vi "3.vi"(8 "Error In":errorcluster, 11 "buffer in":cluster{"Pipe in":i32, "Pipe out":i32}) -> (0 "Error Out":errorcluster, 2 "lectura":bool[](array[boolean]), 3 "buffer out":cluster{"Pipe in":i32, "Pipe out":i32})   [LabVIEW 2016]
uses:
  microchip_solutions_v2013-06-15/USB/Tools/MCHPUSB Custom Driver/Mpusbapi/Dll/Borland_C/Source/mpusbapi.dll
panel:
  out "pLength":i32
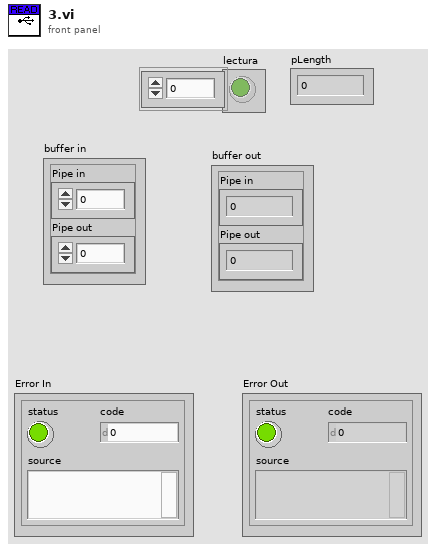
[diagram p1: front panel]
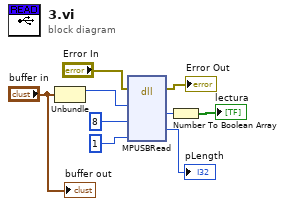
[diagram p0: block diagram]
diagram:
  n1 = Unbundle("buffer in") -> ("Pipe in"=w6:i32)  [unwired: 1 out]
  n2 = dll-call lib="C:/microchip_solutions_v2013-06-15/USB/Tools/MCHPUSB Custom Driver/Mpusbapi/Dll/Borland_C/Source/mpusbapi.dll" fn="MPUSBRead"(error in="Error In", "Pipe in"=w6, "dwLen"=8, "dwMilliseconds"=1) -> (error out=→"Error Out":errorcluster, "pData"=w7:u8, "pLength"=→"pLength":i32)  [unwired: 8 in, 1 out]
  n3 = Number To Boolean Array(number=w7) -> (Boolean array=→"lectura":bool[])
  "buffer out" <- "buffer in"
